vi "Tell Self.vi"(4 "Priority":bool, 7 "Actor in":refnum<class "Actor.lvclass">, 8 "Error in":errorcluster) -> (0 "Error out":errorcluster, 5 "Actor out":refnum<class "Actor.lvclass">)   [LabVIEW 2020, in "jettl.lvlib" / "Stop jettl Msg.lvlib" / "Stop.lvlib"]
uses:
  Stop.lvlib
  Actor/Actor.lvclass
  jettl.lvlib
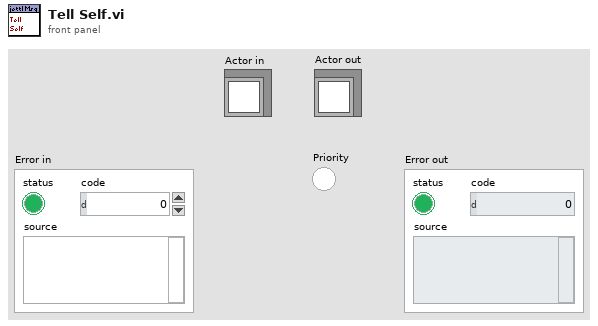
[diagram p1: front panel]
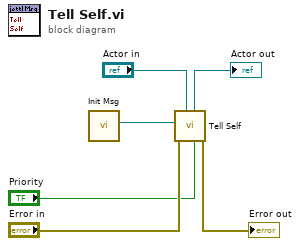
[diagram p0: block diagram]
diagram:
  n1 = call "Init Msg.vi"() -> ("Msg"=w2:refnum<class "Msg.lvclass">)  [unwired: 11 in]
  n2 = call "Tell Self.vi"("Priority"="Priority", "Actor in"="Actor in", "Error in"="Error in", "Msg"=w2) -> ("Error out"=→"Error out":errorcluster, "Actor out"=→"Actor out":refnum<class "Actor.lvclass">)  [unwired: 6 in]
